vi "Data Query.vi"() -> ()   [LabVIEW 2019]
uses:
  <vilib>/addons/database/Connection.llb/DB Tools Open Connec (String).vi
  <vilib>/addons/database/_DB Variant To Data/Database Variant To Data.xnode
  <vilib>/addons/database/NI_Database_API.lvlib
panel:
  out "data 2":string[][](array[string])
  out "data":variant[][](array[variant])
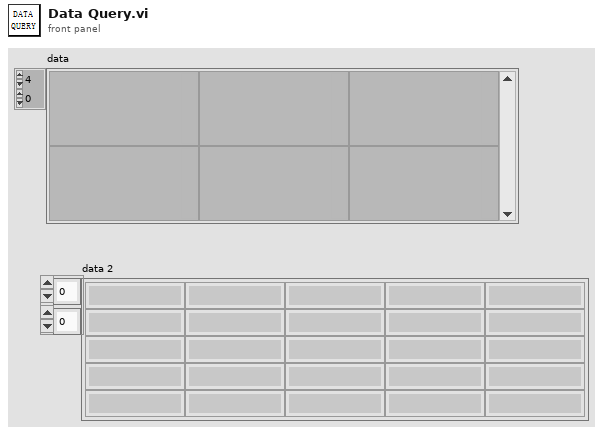
[diagram p1: front panel]
types:
  T1 = typedef "NI_Database_API.lvlib/Conn ObjectReference.ctl" = refnum<k1>
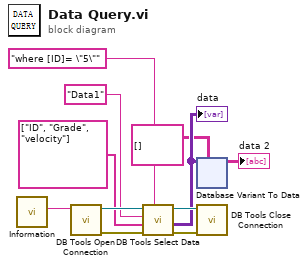
[diagram p0: block diagram]
diagram:
  n1 = call "Information.vi"() -> ("Connection Info"=w7:string)  [unwired: 11 in]
  n2 = call-poly <vilib>:"DB Tools Open Connection.vi"("connection information"=w7) -> ("error out"=w8:errorcluster, "connection reference"=w11:T1)  [unwired: 7 in]
  n3 = call <vilib>:"DB Tools Select Data.vi"("condition"="where [ID]= \"5\"", "error in (no error)"=w8, "columns"=string[] ["ID", "Grade", "velocity"], "table"="Data1", "connection reference"=w11) -> ("error out"=w9:errorcluster, "data"=w3:variant[][], "connection reference out"=w10:T1)  [unwired: 1 in]
  "data" <- w3
  n4 = xnode "Database Variant To Data"("database variant"=w3, "type"=string[][] []) -> ("data"=→"data 2":string[][])  [unwired: 1 in, 1 out]
  n5 = call <vilib>:"DB Tools Close Connection.vi"("error in (no error)"=w9, "connection reference"=w10) -> ()  [unwired: 5 in, 1 out]
